vi "ReadCurrentInfo.vi"(8 "Error In":errorcluster, 11 "reference in":refnum<class "MediaPlayer.lvclass">) -> (0 "Error Out":errorcluster, 2 "Current Info":T1, 3 "reference out":refnum<class "MediaPlayer.lvclass">)   [LabVIEW 2024, in "MediaPlayer.lvclass"]
uses:
  MediaPlayer.lvclass
  MediaPlayer.lvclass/MediaPlayer.ctl
panel:
  # "Connector Pane"
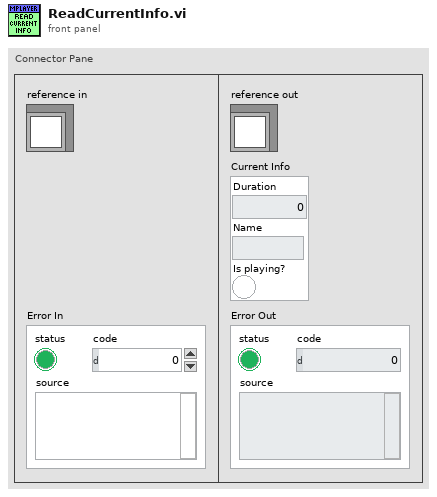
[diagram p1: front panel]
types:
  T1 = cluster{"Duration":dbl, "Name":string, "Is playing?":bool}
  T2 = typedef "MediaPlayer.lvclass/ObjectAttributes.ctl" = cluster{"MediaPlayerData":T3, "Current Info":cluster{"Duration":dbl, "Name":string, "Is playing?":bool}}
  T3 = typedef "MediaPlayer.lvclass/MediaPlayer Data.ctl" = cluster{"Music List":path[], "Current Music Index":u16, "Song Handler":T4, "Device ID":u32}
  T4 = typedef "Sound Output Task ID.ctl" = u32
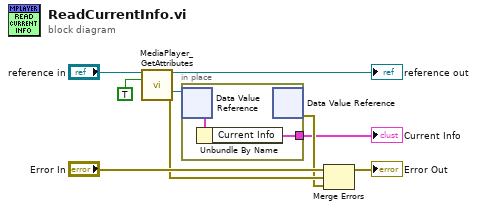
[diagram p0: block diagram]
diagram:
  n1 = call "MediaPlayer_GetAttributes.vi"("reference in"="reference in", "OnlyGetDvrReference(False)"=TRUE) -> ("reference out"=→"reference out":refnum<class "MediaPlayer.lvclass">, "DataRef"=w2:refnum<data-value>, "Error Out"=w8:errorcluster)  [unwired: 10 in, 1 out]
  n2 = in-place {
    in-place-border: [w11] -> w1
    n3 = in-place-dvr #1(w2) -> (w10:T2)  [unwired: 1 out]
    n4 = Unbundle By Name(w10) -> ("Current Info"=w11:T1)
    n5 = in-place-dvr #1() -> (w6:errorcluster)  [unwired: 1 in, 1 out]
  }
  "Current Info" <- w1
  n6 = Merge Errors("Error In", w8, w6) -> (→"Error Out":errorcluster)
